vi "Unique.vi"(11 "strings in":T1) -> (3 "unique strings out":T1)   [LabVIEW 2023]
uses:
  <extravilib>/ChannelInstances/Stream-str/)Channel.ctl
  <extravilib>/ChannelInstances/Stream-str/Read With Abort.vi
  <extravilib>/ChannelInstances/Stream-str/Write With Abort.vi
  <extravilib>/ChannelInstances/Stream-str/EndpointRead.vi
  <extravilib>/ChannelInstances/Stream-str/Endpoint.vi
  <extravilib>/ChannelInstances/Stream-str/)Channel.vi
  <resource>/ChannelSupport/_ChannelSupport/WaitIfNeeded.vi
  <extravilib>/ChannelInstances/Stream-str.lvlib
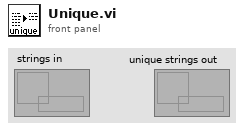
[diagram p1: front panel]
types:
  T1 = typedef "Stream-str.lvlib/)Channel.ctl" = refnum<queue>
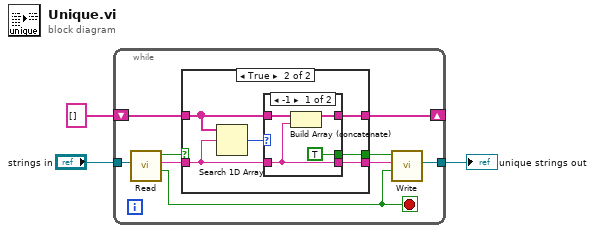
[diagram p0: block diagram]
diagram:
  n1 = while {
    tunnel: [w4] -> w3
    tunnel: "strings in" -> [w9]
    shift-right: [w12] -> _
    shift-left: string[] [] -> [w11]
    stop <- w5 stop-if-true
    n2 = call <extravilib>:"Read.vi"("channel"=w9) -> ("last element?"=w5:bool, "element"=w8:string, "element valid?"=w7:bool)  [unwired: 6 in, 2 out]
    n3 = case shown="True" w7 {
      tunnel: [w14 w19] -> w12
      tunnel: w11 -> [w14 w18]
      tunnel: w8 -> [w13 w17]
      tunnel: [w13 w16] -> w10
      tunnel: [_ w15] -> w6
      frame False {
      }
      frame True {
        n4 = Search 1D Array(1D array=w18, element=w17) -> (index of element=w20:i32)  [unwired: 1 in]
        n5 = case shown="-1" w20 {
          tunnel: w17 -> [w22 _]
          tunnel: [w24 w25] -> w19
          tunnel: w18 -> [w23 w25]
          tunnel: [w22 _] -> w16
          tunnel: [TRUE _] -> w15
          frame -1 {
            n6 = Build Array (concatenate)(w23, w22) -> (w24:string[])
          }
          frame Default {
          }
        }
      }
    }
    n7 = call <extravilib>:"Write.vi"("last element? (F)"=w5, "element"=w10, "element valid? (T)"=w6) -> ("channel"=w4:T1)  [unwired: 6 in, 2 out]
  }
  "unique strings out" <- w3
